vi "ReversedEngineering GetSelectorCaseStates.vi"(1 "StateMachineCaseSelector":refnum<vi>, 5 "error out 2":errorcluster) -> (15 "SelStrings":string[](array[string]), 16 "StateStrings":string[](array[string]), 17 "Frames[]":refnum<vi>[](array[refnum]), 19 "error out":errorcluster)   [LabVIEW 2014]
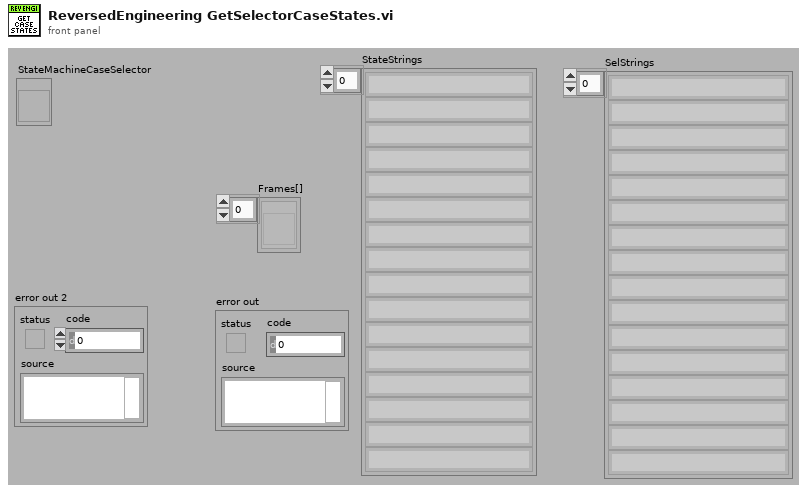
[diagram p1: front panel]
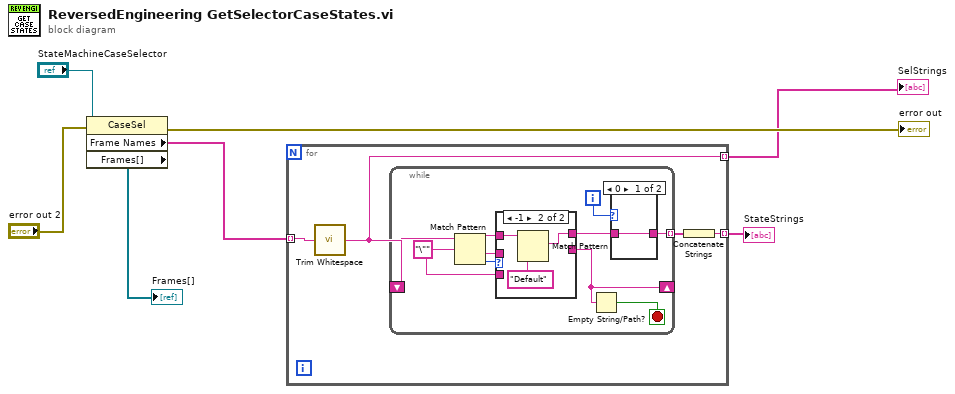
[diagram p0: block diagram]
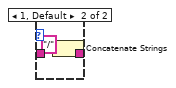
[diagram p2: hidden frame]
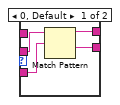
[diagram p3: hidden frame]
diagram:
  n1 = property class="CaseSel"(reference="StateMachineCaseSelector", error in="error out 2") -> (error out=→"error out":errorcluster, "Frame Names"=w2:string[], "Frames[]"=→"Frames[]":refnum<vi>[])  [unwired: 1 out]
  n2 = for {
    tunnel: w2 -> [w9] mode=indexing
    tunnel: [w10] -> w3 mode=indexing
    tunnel: [w8] -> w1 mode=indexing
    n3 = call <vilib>:"Trim Whitespace.vi"("string"=w9) -> ("trimmed string"=w8:string)  [unwired: 1 in]
    n4 = while {
      tunnel: [w15] -> w11 mode=indexing
      shift-right: [w13] -> _
      shift-left: w8 -> [w14]
      i -> [w17]
      stop <- w12 stop-if-true
      w20 = "\"" ("regular expression")
      n5 = Match Pattern(string=w14, regular expression=w20) -> (before substring=w19:string, after substring=w21:string, offset past match=w18:i32)  [unwired: 2 out]
      n6 = case shown="-1" w18 {
        tunnel: w21 -> [w29 _]
        tunnel: w20 -> [w28 _]
        tunnel: [w27 w30] -> w16
        tunnel: w19 -> [_ w32]
        tunnel: [w26 _] -> w13
        frame 0, Default {
          n7 = Match Pattern(string=w29, regular expression=w28) -> (before substring=w27:string, after substring=w26:string)  [unwired: 3 out]
        }
        frame -1 {
          n8 = Match Pattern(string=w32, regular expression="Default") -> (match substring=w30:string)  [unwired: 4 out]
        }
      }
      n9 = Empty String/Path?(string/path=w13) -> (empty?=w12:bool)
      n10 = case shown="0" w17 {
        tunnel: w16 -> [w22 w24]
        tunnel: [w22 w25] -> w15
        frame 0 {
        }
        frame 1, Default {
          n11 = Concatenate Strings("/" ("string"), w24) -> (w25:string)
        }
      }
    }
    n12 = Concatenate Strings(w11) -> (w10:string)
  }
  "SelStrings" <- w1
  "StateStrings" <- w3
